vi "outputCanFileArray.vi"(8 "error in":errorcluster, 11 "interpretedIniFileContentArray":string[](array[string])) -> (0 "error out":errorcluster, 3 "testCaseInCanFileArr":string[](array[string]))   [LabVIEW 2010]
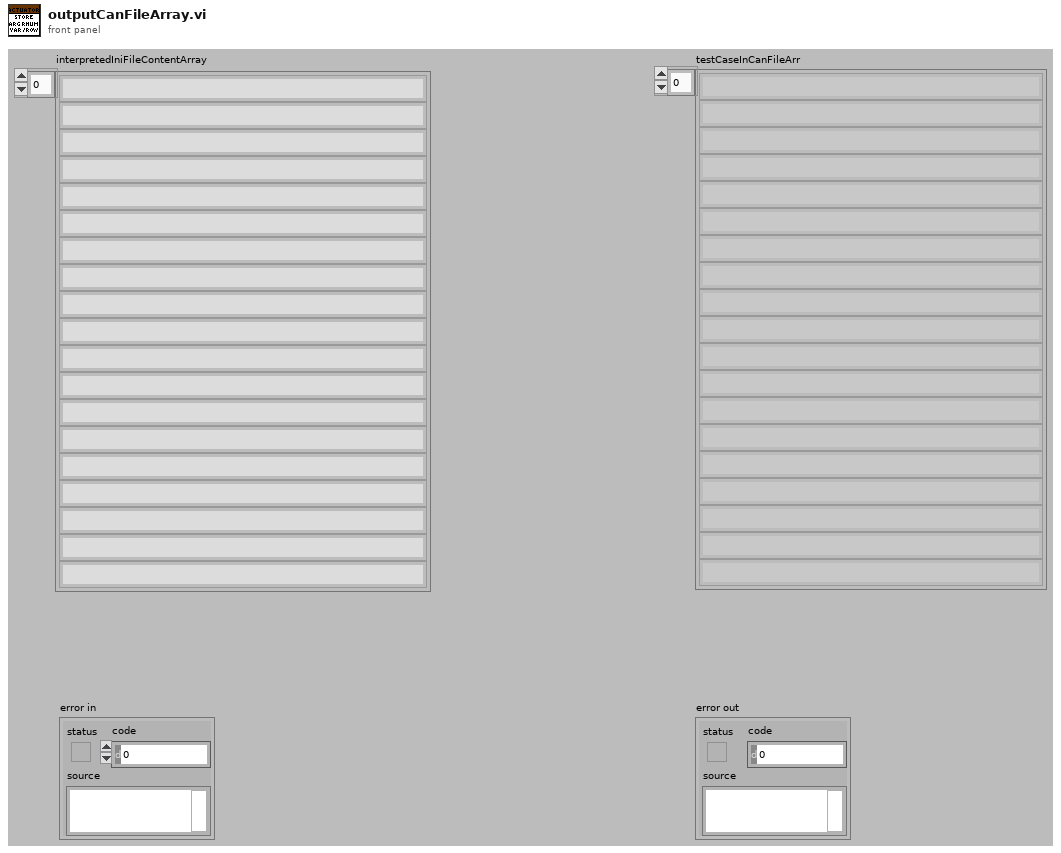
[diagram p1: front panel]
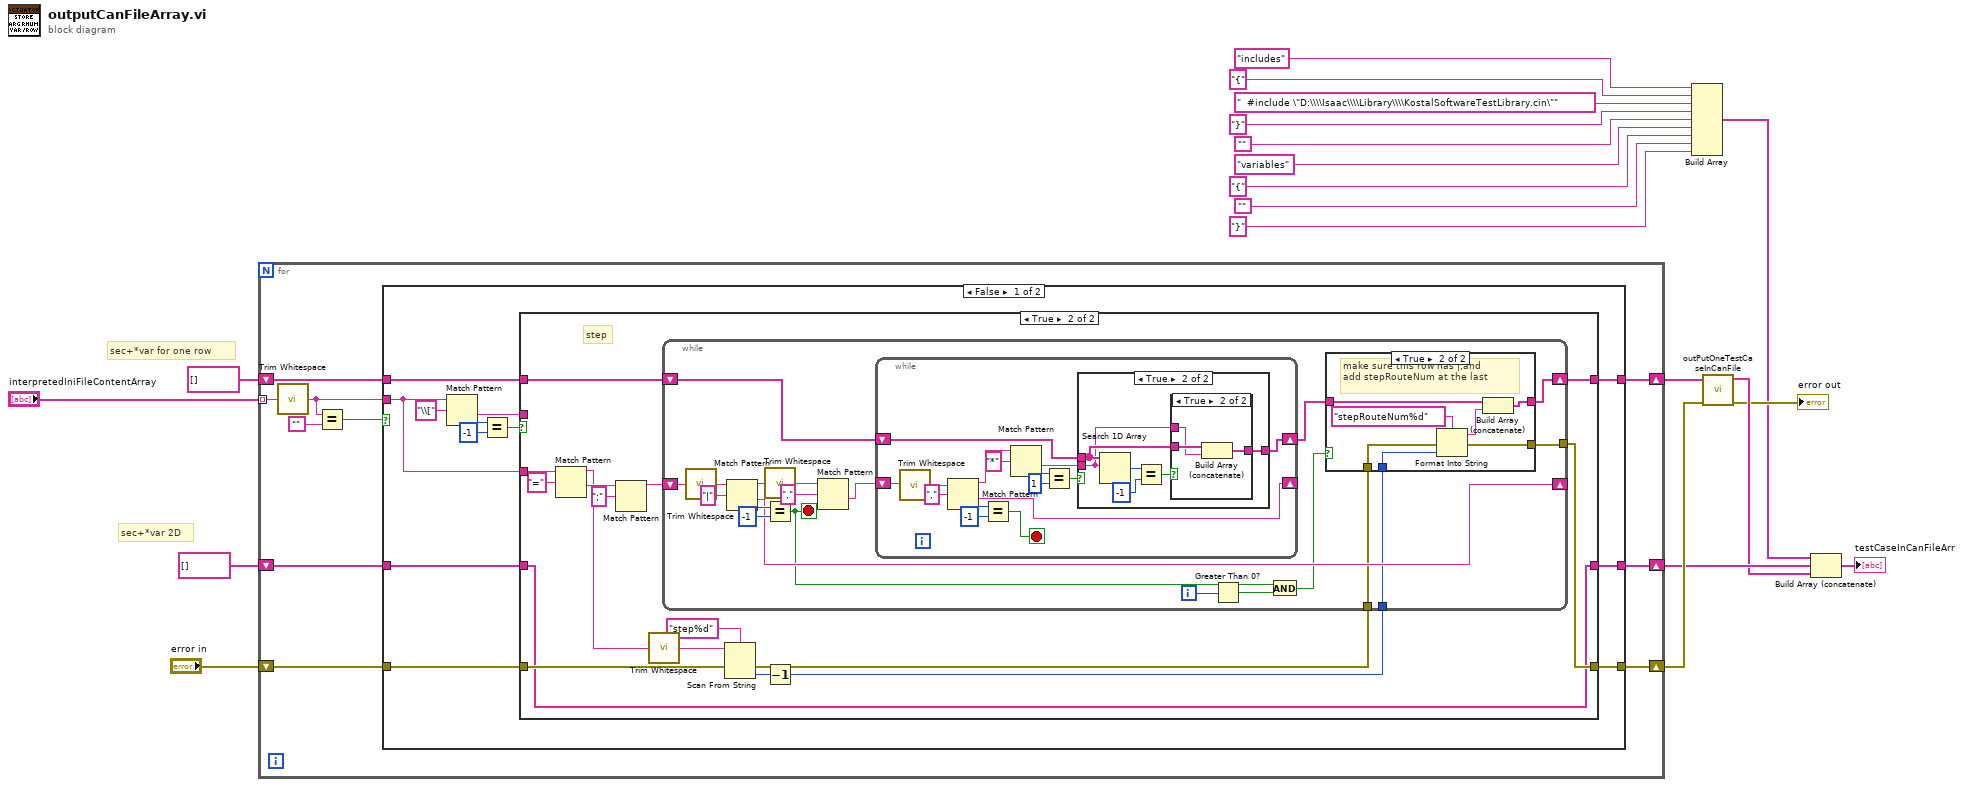
[diagram p0: block diagram]
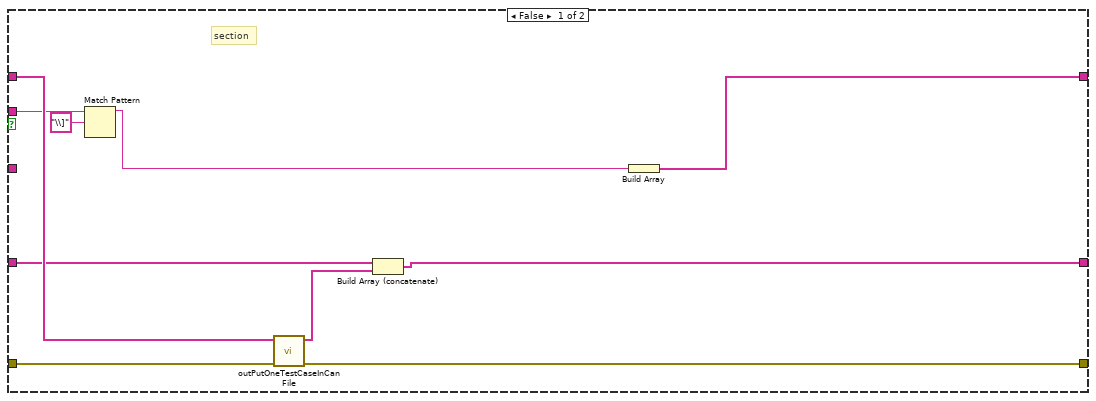
[diagram p2: hidden frame]
diagram:
  # "sec+*var 2D"
  # "sec+*var for one row"
  n1 = for {
    tunnel: "interpretedIniFileContentArray" -> [w30] mode=indexing
    shift-right: [w28] -> w16
    shift-left: string[] [] -> [w29]
    shift-right: [w26] -> w15
    shift-left: "error in" -> [w27]
    shift-right: [w24] -> w14
    shift-left: string[] [] -> [w25]
    n2 = call <vilib>:"Trim Whitespace.vi"("string"=w30) -> ("trimmed string"=w23:string)  [unwired: 1 in]
    n3 = Equal?(x=w23, y="") -> (x = y?=w21:bool)
    n4 = case shown="False" w21 {
      tunnel: w29 -> [w38 w126]
      tunnel: [w37 w126] -> w28
      tunnel: w27 -> [w36 w124]
      tunnel: [w35 w124] -> w26
      tunnel: w25 -> [w34 w125]
      tunnel: [w33 w125] -> w24
      tunnel: w23 -> [w31 _]
      frame False {
        n5 = Match Pattern(string=w31, regular expression="\\[") -> (after substring=w32:string, offset past match=w41:i32)  [unwired: 1 in, 2 out]
        n6 = Equal?(x=w41, y=-1) -> (x = y?=w39:bool)
        n7 = case shown="True" w39 {
          tunnel: w31 -> [_ w67]
          tunnel: w38 -> [w49 w63]
          tunnel: [w52 w53] -> w37
          tunnel: w36 -> [w51 w56]
          tunnel: [w50 w55] -> w35
          tunnel: w34 -> [w48 w54]
          tunnel: [w46 w54] -> w33
          tunnel: w32 -> [w45 _]
          frame False {
            # "section"
            n8 = Match Pattern(string=w45, regular expression="\\]") -> (before substring=w43:string)  [unwired: 1 in, 3 out]
            n9 = call "outPutOneTestCaseInCanFile.vi"("error in"=w51, "sec+*varNoRepeatArr"=w49) -> ("error out"=w50:errorcluster, "oneTestCaseInCanFile"=w47:string[])  [unwired: 8 in]
            n10 = Build Array (concatenate)(w48, w47) -> (w46:string[])
            n11 = Build Array(w43) -> (w52:string[])
          }
          frame True {
            # "step"
            n12 = Match Pattern(string=w67, regular expression="=") -> (before substring=w62:string, after substring=w66:string)  [unwired: 1 in, 2 out]
            n13 = Match Pattern(string=w66, regular expression=";") -> (before substring=w64:string)  [unwired: 1 in, 3 out]
            n14 = call <vilib>:"Trim Whitespace.vi"("string"=w62) -> ("trimmed string"=w61:string)  [unwired: 1 in]
            n15 = Scan From String(format string="step%d" ("regular expression"), input string=w61, error in=w56) -> (error out=w57:errorcluster, output 1=w59:i32)  [unwired: 2 in, 2 out]
            n16 = Decrement(x=w59) -> (x-1=w58:i32)
            n17 = while {
              shift-right: [w83] -> _
              shift-left: w64 -> [w88]
              tunnel: w58 -> [w73]
              tunnel: w57 -> [w72]
              tunnel: [w70] -> w55
              shift-right: [w69] -> w53
              shift-left: w63 -> [w82]
              i -> [w81]
              stop <- w79 stop-if-true
              n18 = call <vilib>:"Trim Whitespace.vi"("string"=w88) -> ("trimmed string"=w87:string)  [unwired: 1 in]
              n19 = Match Pattern(string=w87, regular expression="|") -> (before substring=w75:string, after substring=w83:string, offset past match=w85:i32)  [unwired: 1 in, 1 out]
              n20 = call <vilib>:"Trim Whitespace.vi"("string"=w75) -> ("trimmed string"=w74:string)  [unwired: 1 in]
              n21 = Equal?(x=w85, y=-1) -> (x = y?=w79:bool)
              n22 = Match Pattern(string=w74, regular expression=",") -> (after substring=w76:string)  [unwired: 1 in, 3 out]
              n23 = while {
                shift-right: [w100] -> _
                shift-left: w76 -> [w102]
                shift-right: [w98] -> w71
                shift-left: w82 -> [w103]
                stop <- w109 stop-if-true
                n24 = call <vilib>:"Trim Whitespace.vi"("string"=w102) -> ("trimmed string"=w101:string)  [unwired: 1 in]
                n25 = Match Pattern(string=w101, regular expression=",") -> (before substring=w99:string, after substring=w100:string, offset past match=w111:i32)  [unwired: 1 in, 1 out]
                n26 = Equal?(x=w111, y=-1) -> (x = y?=w109:bool)
                n27 = Match Pattern(string=w99, regular expression="*") -> (after substring=w104:string, offset past match=w107:i32)  [unwired: 1 in, 2 out]
                n28 = Equal?(x=w107, y=1) -> (x = y?=w105:bool)
                n29 = case shown="True" w105 {
                  tunnel: w104 -> [_ w115]
                  tunnel: w103 -> [w113 w116]
                  tunnel: [w113 w114] -> w98
                  frame False {
                  }
                  frame True {
                    n30 = Search 1D Array(1D array=w116, element=w115) -> (index of element=w119:i32)  [unwired: 1 in]
                    n31 = Equal?(x=w119, y=-1) -> (x = y?=w117:bool)
                    n32 = case shown="True" w117 {
                      tunnel: w116 -> [w120 w123]
                      tunnel: w115 -> [_ w122]
                      tunnel: [w120 w121] -> w114
                      frame False {
                      }
                      frame True {
                        n33 = Build Array (concatenate)(w123, w122) -> (w121:string[])
                      }
                    }
                  }
                }
              }
              n34 = Greater Than 0?(x=w81) -> (x > 0?=w80:bool)
              n35 = And(x=w79, y=w80) -> (x .and. y?=w78:bool)
              n36 = case shown="True" w78 {
                tunnel: w73 -> [_ w96]
                tunnel: w72 -> [w89 w95]
                tunnel: w71 -> [w90 w94]
                tunnel: [w90 w92] -> w69
                tunnel: [w89 w91] -> w70
                frame False {
                }
                frame True {
                  # "make sure this row has |,and \nadd stepRouteNum at the last"
                  n37 = Format Into String(format string="stepRouteNum%d" ("regular expression"), error in=w95, w96) -> (resulting string=w93:string, error out=w91:errorcluster)  [unwired: 1 in]
                  n38 = Build Array (concatenate)(w94, w93) -> (w92:string[])
                }
              }
            }
          }
        }
      }
      frame True {
      }
    }
  }
  n39 = Build Array("includes", "{", "  #include \"D:\\\\Isaac\\\\Library\\\\KostalSoftwareTestLibrary.cin\"", "}", "", "variables", "{", "", "}") -> (w1:string[])
  n40 = call "outPutOneTestCaseInCanFile.vi"("error in"=w15, "sec+*varNoRepeatArr"=w16) -> ("error out"=→"error out":errorcluster, "oneTestCaseInCanFile"=w13:string[])  [unwired: 8 in]
  n41 = Build Array (concatenate)(w1, w14, w13) -> (→"testCaseInCanFileArr":string[])
